vi "Test2.vi"() -> ()   [LabVIEW 2016]
uses:
  <vilib>/Utility/miscctls.llb/LVRectTypeDef.ctl
  <vilib>/picture/picture.llb/imagedata.ctl
  <vilib>/Utility/inputDevices.llb/mouseAcquire.vi
  <vilib>/Utility/inputDevices.llb/closeMouse.vi
  C:/Windows/System32/user32.dll
panel:
  out "Bool 2":i32
  out "Bounds":T1
  out "2D Picture":picture
  out "Bool":i32
  out "return type":i32 format="%x"
  in  "rectClinet":T2
  out "return type 2":i32
  out "point":T2
  in  "stop":bool
  out "Numeric":i32
  out "axis info":T3
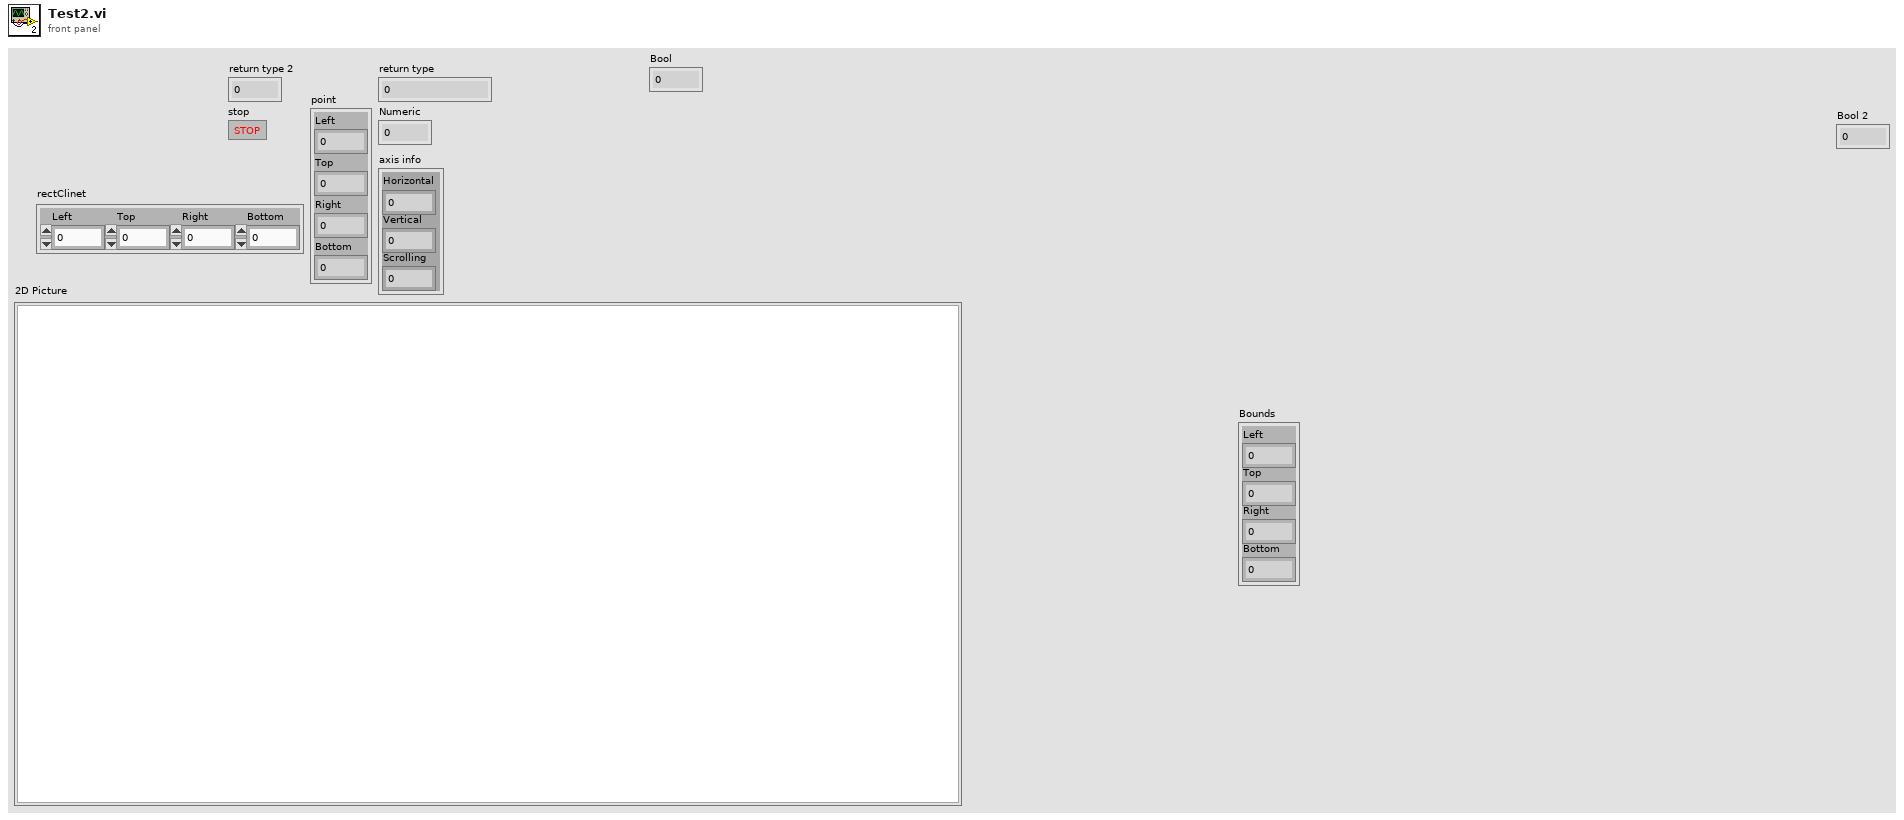
[diagram p1: front panel]
types:
  T1 = typedef "LVRectTypeDef.ctl" = cluster{"Left":i16, "Top":i16, "Right":i16, "Bottom":i16}
  T2 = cluster{"Left":i32, "Top":i32, "Right":i32, "Bottom":i32}
  T3 = cluster{"Horizontal":i32, "Vertical":i32, "Scrolling":i32}
  T4 = typedef "imagedata.ctl" = cluster{"image type":i32, "image depth":i32, "image":u8[], "mask":u8[], "colors":u32[], "Rectangle":cluster{"left":i16, "top":i16, "right":i16, "bottom":i16}}
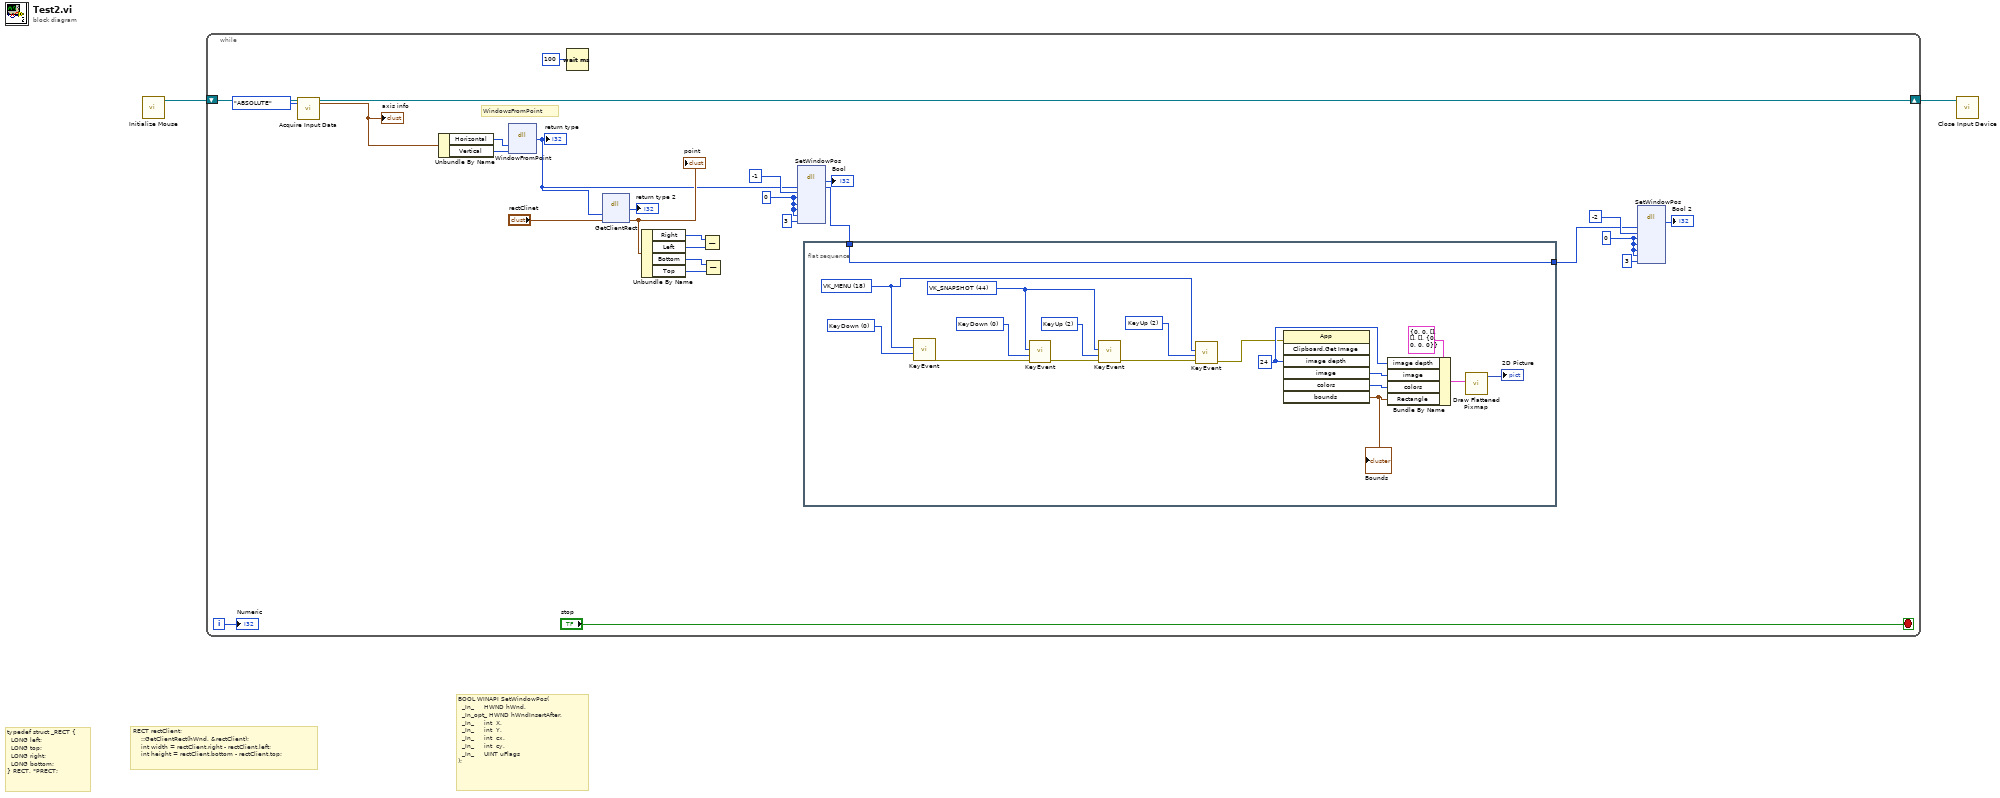
[diagram p0: block diagram]
diagram:
  # "BOOL WINAPI SetWindowPos(\n  _In_     HWND hWnd,\n  _In_opt_ HWND hWndInsertAfter,\n  _In_     int  X,\n  _In_     int  Y,\n  _In_     int  cx,\n  _In_     int  cy,\n  _In_     UINT uFlags\n);"
  # "typedef struct _RECT {\n  LONG left;\n  LONG top;\n  LONG right;\n  LONG bottom;\n} RECT, *PRECT;"
  # "RECT rectClient;  \n    ::GetClientRect(hWnd, &rectClient);  \n    int width = rectClient.right - rectClient.left;  \n    int height = rectClient.bottom - rectClient.top;"
  n1 = call <vilib>:"Initialize Mouse.vi"() -> ("device ID"=w2:refnum<k1>)  [unwired: 10 in, 1 out]
  n2 = while {
    shift-right: [w26] -> w1
    shift-left: w2 -> [w29]
    i -> [w24]
    stop <- "stop" stop-if-true
    w6 = 0 ("X")
    w12 = 0 ("X")
    # "WindowsFromPoint"
    n3 = call-poly <vilib>:"Acquire Input Data.vi"("device ID"=w29, "key mode"=enum16{"RELATIVE", "ABSOLUTE"}."ABSOLUTE") -> ("device ID"=w26:refnum<k1>, "axis info"=w27:T3)  [unwired: 14 in, 2 out]
    "axis info" <- w27
    n4 = Unbundle By Name(w27) -> ("Horizontal"=w22:i32, "Vertical"=w21:i32)
    n5 = dll-call lib="C:/Windows/System32/user32.dll" fn="WindowFromPoint"("x"=w22, "y"=w21) -> ("return type"=w3:i32)  [unwired: 5 in, 2 out]
    "return type" <- w3
    n6 = Wait (ms)(milliseconds to wait=u32 100) -> ()  [unwired: 1 out]
    n7 = dll-call lib="C:/Windows/System32/user32.dll" fn="GetClientRect"("HWND"=w3, "point"="rectClinet") -> ("return type"=→"return type 2":i32, "point"=w18:T2)  [unwired: 4 in, 2 out]
    "point" <- w18
    n8 = Unbundle By Name(w18) -> ("Right"=w16:i32, "Left"=w17:i32, "Bottom"=w15:i32, "Top"=w14:i32)
    n9 = Subtract(x=w16, y=w17) -> ()  [unwired: 1 out]
    n10 = Subtract(x=w15, y=w14) -> ()  [unwired: 1 out]
    n11 = dll-call lib="C:/Windows/System32/user32.dll" fn="SetWindowPos"("HWND"=w3, "HWNDInsertAfter"=-1, "X"=w12, "Y"=w12, "cx"=w12, "cy"=w12, "Flag"=u32 3) -> ("Bool"=→"Bool":i32, "HWND"=w9:i32)  [unwired: 9 in, 2 out]
    n12 = flat-sequence {
      tunnel: w9 -> [w40]
      tunnel: [w40] -> w4
      frame #0 {
        w35 = u8 44 items=["Undefined", "VK_LBUTTON", "VK_RBUTTON", "VK_CANCEL", "VK_MBUTTON", "VK_XBUTTON1", "VK_XBUTTON2", "Undefined", "VK_BACK", "VK_TAB", "Reserved", "Reserved", "VK_CLEAR", "VK_RETURN", "Undefined", "Undefined", "VK_SHIFT", "VK_CONTROL", "VK_MENU", "VK_PAUSE", "VK_CAPITAL", "VK_KANA", "Undefined", "VK_JUNJA", "VK_FINAL", "VK_HANJA", "Undefined", "VK_ESCAPE", "VK_CONVERT", "VK_NONCONVERT", "VK_ACCEPT", "VK_MODECHANGE", "VK_SPACE", "VK_PRIOR", "VK_NEXT", "VK_END", "VK_HOME", "VK_LEFT", "VK_UP", "VK_RIGHT", "VK_DOWN", "VK_SELECT", "VK_PRINT", "VK_EXECUTE", "VK_SNAPSHOT", "VK_INSERT", "VK_DELETE", "VK_HELP", "VK_0", "VK_1", "VK_2", "VK_3", "VK_4", "VK_5", "VK_6", "VK_7", "VK_8", "VK_9", "Undefined", "Undefined", "Undefined", "Undefined", "Undefined", "Undefined", "Undefined", "VK_A", "VK_B", "VK_C", "VK_D", "VK_E", "VK_F", "VK_G", "VK_H", "VK_I", "VK_J", "VK_K", "VK_L", "VK_M", "VK_N", "VK_O", "VK_P", "VK_Q", "VK_R", "VK_S", "VK_T", "VK_U", "VK_V", "VK_W", "VK_X", "VK_Y", "VK_Z", "VK_LWIN", "VK_RWIN", "VK_APPS", "Reserved", "VK_SLEEP", "VK_NUMPAD0", "VK_NUMPAD1", "VK_NUMPAD2", "VK_NUMPAD3", "VK_NUMPAD4", "VK_NUMPAD5", "VK_NUMPAD6", "VK_NUMPAD7", "VK_NUMPAD8", "VK_NUMPAD9", "VK_MULTIPLY", "VK_ADD", "VK_SEPARATOR", "VK_SUBTRACT", "VK_DECIMAL", "VK_DIVIDE", "VK_F1", "VK_F2", "VK_F3", "VK_F4", "VK_F5", "VK_F6", "VK_F7", "VK_F8", "VK_F9", "VK_F10", "VK_F11", "VK_F12", "VK_F13", "VK_F14", "VK_F15", "VK_F16", "VK_F17", "VK_F18", "VK_F19  ", "VK_F20 ", "VK_F21", "VK_F22 ", "VK_F23", "VK_F24", "Unsigned", "Unsigned", "Unsigned", "Unsigned", "Unsigned", "Unsigned", "Unsigned", "Unsigned", "VK_NUMLOCK", "VK_SCROLL", "OEM Specific", " OEM Speicfic", "OEM Speicfic", "OEM Specific", "OEM Specific", "Unassigned", "Unassigned", "Unassigned", "Unassigned", "Unassigned", "Unassigned", "Unassigned", "Unassigned", "Unassigned", "VK_LSHIFT", "VK_RSHIFT", "VK_LCONTROL", "VK_RCONTROL", "VK_LMENU", "VK_RMENU", "VK_BROWSER_BACK", "VK_BROWSER_FORWARD", "VK_BROWSER_REFRESH", "VK_BROWSER_STOP", "VK_BROWSER_SEARCH", "VK_BROWSER_FAVORITES ", "VK_BROWSER_HOME", "VK_VOLUME_MUTE", "VK_VOLUME_DOWN", "VK_VOLUME_UP", "VK_MEDIA_NEXT_TRACK", "VK_MEDIA_PREV_TRACK", "VK_MEDIA_STOP ", "VK_MEDIA_PLAY_PAUSE", "VK_LAUNCH_MAIL", "VK_LAUNCH_MEDIA_SELECT", "VK_LAUNCH_APP1", "VK_LAUNCH_APP2", "Reserved", "Reserved", "VK_OEM_1(;:)", "VK_OEM_PLUS(+) ", "VK_OEM_COMMA(,)", "VK_OEM_MINUS(-)", "VK_OEM_PERIOD(.)", "VK_OEM_2(/?)", "VK_OEM_3(~`)", "Reserved", "Reserved", "Reserved", "Reserved", "Reserved", "Reserved", "Reserved", "Reserved", "Reserved", "Reserved", "Reserved", "Reserved", "Reserved", "Reserved", "Reserved", "Reserved", "Reserved", "Reserved", "Reserved", "Reserved", "Reserved", "Reserved", "Reserved", "Reserved", "Reserved", "Reserved", "VK_OEM_4 ([{)", "VK_OEM_5 (\\|)", "VK_OEM_6 (]})", "VK_OEM_7 ('\")", "VK_OEM_8", "Reserved", "Reserved", "VK_OEM_102", "OEM Specific", "OEM Specific", "VK_PROCESSKEY", "OEM Specific", "VK_PACKET", "Unassigned", "OEM Specific", "OEM Specific", "OEM Specific", "OEM Specific", "OEM Specific", "OEM Specific", "OEM Specific", "OEM Specific", "OEM Specific", "OEM Specific", "OEM Specific", "OEM Specific", "OEM Specific", "VK_ATTN", "VK_CRSEL", "VK_EXSEL", "VK_EREOF", "VK_PLAY", "VK_ZOOM", "VK_NONAME", "VK_PA1", "VK_OEM_CLEAR "] ("VK_CODE")
        w32 = u32 2 items=["KeyDown"=0, "KeyUp"=2] ("Option")
        w39 = u32 0 items=["KeyDown"=0, "KeyUp"=2] ("Option")
        w34 = u32 2 items=["KeyDown"=0, "KeyUp"=2] ("Option")
        w38 = u32 0 items=["KeyDown"=0, "KeyUp"=2] ("Option")
        w43 = 24 ("Image Depth")
        w31 = u8 18 items=["Undefined", "VK_LBUTTON", "VK_RBUTTON", "VK_CANCEL", "VK_MBUTTON", "VK_XBUTTON1", "VK_XBUTTON2", "Undefined", "VK_BACK", "VK_TAB", "Reserved", "Reserved", "VK_CLEAR", "VK_RETURN", "Undefined", "Undefined", "VK_SHIFT", "VK_CONTROL", "VK_MENU", "VK_PAUSE", "VK_CAPITAL", "VK_KANA", "Undefined", "VK_JUNJA", "VK_FINAL", "VK_HANJA", "Undefined", "VK_ESCAPE", "VK_CONVERT", "VK_NONCONVERT", "VK_ACCEPT", "VK_MODECHANGE", "VK_SPACE", "VK_PRIOR", "VK_NEXT", "VK_END", "VK_HOME", "VK_LEFT", "VK_UP", "VK_RIGHT", "VK_DOWN", "VK_SELECT", "VK_PRINT", "VK_EXECUTE", "VK_SNAPSHOT", "VK_INSERT", "VK_DELETE", "VK_HELP", "VK_0", "VK_1", "VK_2", "VK_3", "VK_4", "VK_5", "VK_6", "VK_7", "VK_8", "VK_9", "Undefined", "Undefined", "Undefined", "Undefined", "Undefined", "Undefined", "Undefined", "VK_A", "VK_B", "VK_C", "VK_D", "VK_E", "VK_F", "VK_G", "VK_H", "VK_I", "VK_J", "VK_K", "VK_L", "VK_M", "VK_N", "VK_O", "VK_P", "VK_Q", "VK_R", "VK_S", "VK_T", "VK_U", "VK_V", "VK_W", "VK_X", "VK_Y", "VK_Z", "VK_LWIN", "VK_RWIN", "VK_APPS", "Reserved", "VK_SLEEP", "VK_NUMPAD0", "VK_NUMPAD1", "VK_NUMPAD2", "VK_NUMPAD3", "VK_NUMPAD4", "VK_NUMPAD5", "VK_NUMPAD6", "VK_NUMPAD7", "VK_NUMPAD8", "VK_NUMPAD9", "VK_MULTIPLY", "VK_ADD", "VK_SEPARATOR", "VK_SUBTRACT", "VK_DECIMAL", "VK_DIVIDE", "VK_F1", "VK_F2", "VK_F3", "VK_F4", "VK_F5", "VK_F6", "VK_F7", "VK_F8", "VK_F9", "VK_F10", "VK_F11", "VK_F12", "VK_F13", "VK_F14", "VK_F15", "VK_F16", "VK_F17", "VK_F18", "VK_F19  ", "VK_F20 ", "VK_F21", "VK_F22 ", "VK_F23", "VK_F24", "Unsigned", "Unsigned", "Unsigned", "Unsigned", "Unsigned", "Unsigned", "Unsigned", "Unsigned", "VK_NUMLOCK", "VK_SCROLL", "OEM Specific", " OEM Speicfic", "OEM Speicfic", "OEM Specific", "OEM Specific", "Unassigned", "Unassigned", "Unassigned", "Unassigned", "Unassigned", "Unassigned", "Unassigned", "Unassigned", "Unassigned", "VK_LSHIFT", "VK_RSHIFT", "VK_LCONTROL", "VK_RCONTROL", "VK_LMENU", "VK_RMENU", "VK_BROWSER_BACK", "VK_BROWSER_FORWARD", "VK_BROWSER_REFRESH", "VK_BROWSER_STOP", "VK_BROWSER_SEARCH", "VK_BROWSER_FAVORITES ", "VK_BROWSER_HOME", "VK_VOLUME_MUTE", "VK_VOLUME_DOWN", "VK_VOLUME_UP", "VK_MEDIA_NEXT_TRACK", "VK_MEDIA_PREV_TRACK", "VK_MEDIA_STOP ", "VK_MEDIA_PLAY_PAUSE", "VK_LAUNCH_MAIL", "VK_LAUNCH_MEDIA_SELECT", "VK_LAUNCH_APP1", "VK_LAUNCH_APP2", "Reserved", "Reserved", "VK_OEM_1(;:)", "VK_OEM_PLUS(+) ", "VK_OEM_COMMA(,)", "VK_OEM_MINUS(-)", "VK_OEM_PERIOD(.)", "VK_OEM_2(/?)", "VK_OEM_3(~`)", "Reserved", "Reserved", "Reserved", "Reserved", "Reserved", "Reserved", "Reserved", "Reserved", "Reserved", "Reserved", "Reserved", "Reserved", "Reserved", "Reserved", "Reserved", "Reserved", "Reserved", "Reserved", "Reserved", "Reserved", "Reserved", "Reserved", "Reserved", "Reserved", "Reserved", "Reserved", "VK_OEM_4 ([{)", "VK_OEM_5 (\\|)", "VK_OEM_6 (]})", "VK_OEM_7 ('\")", "VK_OEM_8", "Reserved", "Reserved", "VK_OEM_102", "OEM Specific", "OEM Specific", "VK_PROCESSKEY", "OEM Specific", "VK_PACKET", "Unassigned", "OEM Specific", "OEM Specific", "OEM Specific", "OEM Specific", "OEM Specific", "OEM Specific", "OEM Specific", "OEM Specific", "OEM Specific", "OEM Specific", "OEM Specific", "OEM Specific", "OEM Specific", "VK_ATTN", "VK_CRSEL", "VK_EXSEL", "VK_EREOF", "VK_PLAY", "VK_ZOOM", "VK_NONAME", "VK_PA1", "VK_OEM_CLEAR "] ("VK_CODE")
        n13 = call "KeyEvent.vi"("Option"=w39, "VK_CODE"=w31) -> ("error out"=w37:errorcluster)  [unwired: 9 in]
        n14 = call "KeyEvent.vi"("error in"=w37, "Option"=w38, "VK_CODE"=w35) -> ("error out"=w36:errorcluster)  [unwired: 8 in]
        n15 = call "KeyEvent.vi"("error in"=w36, "Option"=w34, "VK_CODE"=w35) -> ("error out"=w33:errorcluster)  [unwired: 8 in]
        n16 = call "KeyEvent.vi"("error in"=w33, "Option"=w32, "VK_CODE"=w31) -> ("error out"=w30:errorcluster)  [unwired: 8 in]
        n17 = invoke class="App" method="Clipboard.Get Image"(error in=w30, "image depth"=w43) -> ("image"=w44:u8[], "colors"=w45:u32[], "bounds"=w46:T1)  [unwired: 5 in, 4 out]
        "Bounds" <- w46
        n18 = Bundle By Name(cluster=T4 {"image type"=0, "image depth"=0, "image"=[], "mask"=[], "colors"=[], "Rectangle"={"left"=0, "top"=0, "right"=0, "bottom"=0}} ("image data"), "image depth"=w43, "image"=w44, "colors"=w45, "Rectangle"=w46) -> (w41:T4)
        n19 = call <vilib>:"Draw Flattened Pixmap.vi"("image data"=w41) -> ("new picture"=→"2D Picture":picture)  [unwired: 8 in]
      }
    }
    n20 = dll-call lib="C:/Windows/System32/user32.dll" fn="SetWindowPos"("HWND"=w4, "HWNDInsertAfter"=-2, "X"=w6, "Y"=w6, "cx"=w6, "cy"=w6, "Flag"=u32 3) -> ("Bool"=→"Bool 2":i32)  [unwired: 10 in, 2 out]
    "Numeric" <- w24
  }
  n21 = call-poly <vilib>:"Close Input Device.vi"("device ID"=w1) -> ()  [unwired: 9 in, 1 out]
